vi "I2C LCD - Initialize.vi"(10 "Slave Address (7-bit)":u8, 11 "Channel Name":tag) -> (0 "error out":errorcluster, 3 "I2C Ref Out":T1)   [LabVIEW 2017]
uses:
  <vilib>/myRIO/Instrument Drivers/Onboard IO/I2C/typedefs/I2C Reference.ctl
  <vilib>/myRIO/Common/Instrument Driver Framework/Utilities/typedefs/myRIO Generic Hardware Reference.ctl
  <vilib>/myRIO/Common/Instrument Driver Framework/Utilities/typedefs/Hardware Version Enum.ctl
  <vilib>/myRIO/Common/Instrument Driver Framework/Utilities/typedefs/myRIO v1.0 Reference.ctl
  <vilib>/myRIO/Common/Instrument Driver Framework/Utilities/typedefs/Generic FPGA Reference.ctl
  <vilib>/myRIO/Common/Instrument Driver Framework/myRIO v1.0/I2C/typedefs/I2C Channels Enum.ctl
  <vilib>/myRIO/Instrument Drivers/Onboard IO/I2C/typedefs/I2C Configuration.ctl
  <vilib>/myRIO/Instrument Drivers/Onboard IO/I2C/typedefs/I2C Transfer Rate.ctl
  <vilib>/myRIO/Instrument Drivers/Onboard IO/I2C/typedefs/I2C User Configuration.ctl
  <vilib>/Utility/error.llb/Error Cluster From Error Code.vi
  <vilib>/myRIO/Common/Instrument Driver Framework/myRIO v1.0/I2C/vis/myRIO v1.0 Configure I2C.vi
  <vilib>/myRIO/Instrument Drivers/Onboard IO/I2C/I2C.lvlib
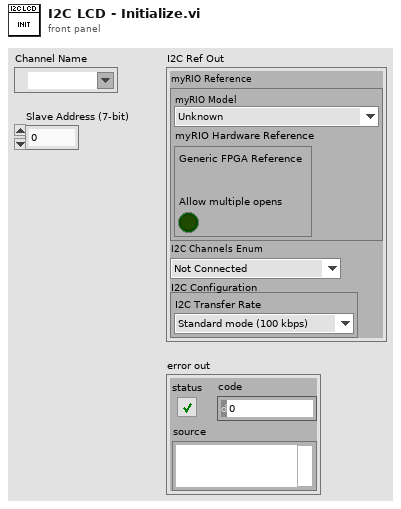
[diagram p1: front panel]
types:
  T1 = typedef "I2C.lvlib/I2C Reference.ctl" = cluster{"myRIO Reference":T2, "I2C Channels Enum":T6, "I2C Configuration":T7}
  T2 = typedef "myRIO Generic Hardware Reference.ctl" = cluster{"myRIO Model":T3, "myRIO Hardware Reference":T4}
  T3 = typedef "Hardware Version Enum.ctl" = enum16{"Unknown", "myRIO-1900", "myRIO-1950", "roboRIO", "NI ELVIS RIO CM"}
  T4 = typedef "myRIO v1.0 Reference.ctl" = cluster{"Generic FPGA Reference":T5, "Allow multiple opens":bool}
  T5 = typedef "Generic FPGA Reference.ctl" = refnum<k20>
  T6 = typedef "I2C Channels Enum.ctl" = enum16{"Not Connected", "A/I2C", "B/I2C", "I2C/I2C"}
  T7 = typedef "I2C.lvlib/I2C Configuration.ctl" = cluster{"I2C Transfer Rate":T8}
  T8 = typedef "I2C.lvlib/I2C Transfer Rate.ctl" = enum16{"Standard mode (100 kbps)", "Fast mode (400 kbps)"}
  T9 = typedef "I2C.lvlib/I2C User Configuration.ctl" = cluster{"I2C Transfer Rate":T8}
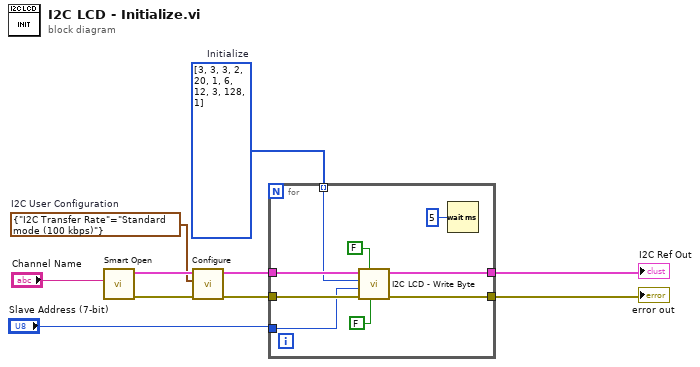
[diagram p0: block diagram]
diagram:
  w9 = u8[] [3, 3, 3, 2, 20, 1, 6, 12, 3, 128, 1]  # Initialize
  w2 = T9 {"I2C Transfer Rate"=enum."Standard mode (100 kbps)"}  # I2C User Configuration
  n1 = call <vilib>:"Smart Open.vi"("Channel Name"="Channel Name") -> ("error out"=w4:errorcluster, "I2C Ref Out"=w3:T1)  [unwired: 9 in]
  n2 = call <vilib>:"Configure.vi"("error in (no error)"=w4, "I2C User Configuration"=w2, "I2C Ref In"=w3) -> ("error out"=w5:errorcluster, "I2C Ref Out"=w6:T1)  [unwired: 7 in]
  n3 = for {
    tunnel: w5 -> [w15]
    tunnel: w6 -> [w16]
    tunnel: "Slave Address (7-bit)" -> [w14]
    tunnel: [w18] -> w10
    tunnel: [w17] -> w7
    tunnel: w9 -> [w13] mode=indexing
    n4 = call "I2C LCD - Write Byte.vi"("BL"=FALSE, "RS"=FALSE, "error in (no error)"=w15, "Slave Address (7-bit)"=w14, "Numeric"=w13, "I2C Ref"=w16) -> ("error out"=w17:errorcluster, "I2C Ref Out"=w18:T1)  [unwired: 4 in]
    n5 = Wait (ms)(milliseconds to wait=u32 5) -> ()  [unwired: 1 out]
  }
  "I2C Ref Out" <- w10
  "error out" <- w7
